vi "Do.vi"(8 "error in (no error)":errorcluster, 10 "Actor in":refnum<class "Actor.lvclass">, 11 "Results from Cam 1 Msg":refnum<class "Results from Cam 1 Msg.lvclass">) -> (0 "error out":errorcluster, 2 "Actor out":refnum<class "Actor.lvclass">)   [LabVIEW 2014, in "Results from Cam 1 Msg.lvclass"]
doc: "This VI delivers the message to the actor by calling the appropriate method(s) on the actor."
uses:
  Results from Cam 1 Msg.lvclass
  <vilib>/ActorFramework/Actor/Actor.lvclass
  HIJ 4 Alignment Cams App/HIJ 4 Alignment Cams App.lvclass
  Abstract Messages/Publish Analyze Results Msg/Publish Analyze Results Msg.lvclass/Publish Analyze Results Msg.ctl
  Abstract Messages/Publish Analyze Results Msg/Publish Analyze Results Msg.lvclass
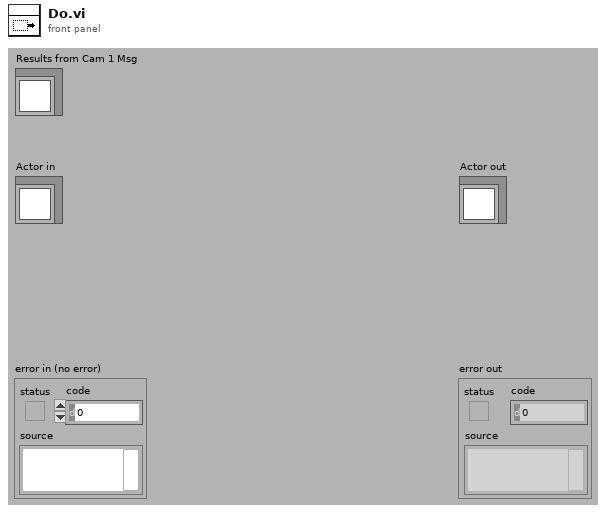
[diagram p1: front panel]
types:
  T1 = cluster{"Image Nr.":i32, "Results":refnum<class "Analyze Results Base.lvclass">[], "Parameters":refnum<class "Analyze Parameter Base.lvclass">[]}
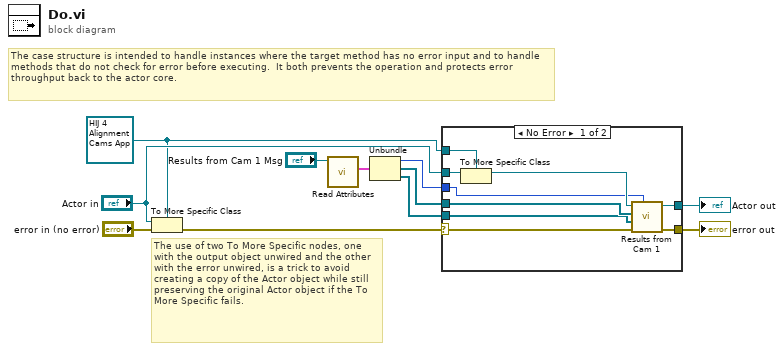
[diagram p0: block diagram]
diagram:
  w6 = refnum<class "HIJ 4 Alignment Cams App.lvclass"> refnum ("Actor in")
  # "The use of two To More Specific nodes, one with the output object unwired and the other with the error unwired, is a trick to avoid creating a copy of the Actor object while still preserving the original Actor object if the To More Specific fails."
  # "The case structure is intended to handle instances where the target method has no error input and to handle methods that do not check for error before executing.  It both prevents the operation and protects error throughput back to the actor core."
  n1 = To More Specific Class(target class=w6, reference="Actor in", error in="error in (no error)") -> (error out=w10:errorcluster)  [unwired: 1 out]
  n2 = call "Read Attributes.vi"("Abstract Message Template in"="Results from Cam 1 Msg") -> ("Payload"=w4:T1)  [unwired: 9 in, 1 out]
  n3 = Unbundle(w4) -> ("Image Nr."=w3:i32, "Results"=w2:refnum<class "Analyze Results Base.lvclass">[], "Parameters"=w1:refnum<class "Analyze Parameter Base.lvclass">[])
  n4 = case shown="No Error" w10 {
    selector: w10 -> [w18 w22]
    tunnel: [w20 w22] -> w9
    tunnel: [w19 w21] -> w8
    tunnel: "Actor in" -> [w17 w21]
    tunnel: w6 -> [w16 _]
    tunnel: w3 -> [w14 _]
    tunnel: w2 -> [w13 _]
    tunnel: w1 -> [w12 _]
    frame No Error {
      n5 = To More Specific Class(target class=w16, reference=w17) -> (specific class reference=w15:refnum<class "HIJ 4 Alignment Cams App.lvclass">)  [unwired: 1 in, 1 out]
      n6 = call "Results from Cam 1.vi"("Image Nr."=w14, "error in (no error)"=w18, "Parameters"=w12, "Results"=w13, "HIJ Multiple Cams App Demo in"=w15) -> ("error out"=w20:errorcluster, "HIJ Multiple Cams App Demo out"=w19:refnum<class "HIJ 4 Alignment Cams App.lvclass">)  [unwired: 5 in]
    }
    frame Error {
      # "If type check fails, pass the original object out again."
    }
  }
  "error out" <- w9
  "Actor out" <- w8
